vi "picturebox.vi"(8 "s":string, 11 "PictureBox":refnum<k24>(container)) -> ()   [LabVIEW 2024]
uses:
  System.Drawing
  System.Windows.Forms
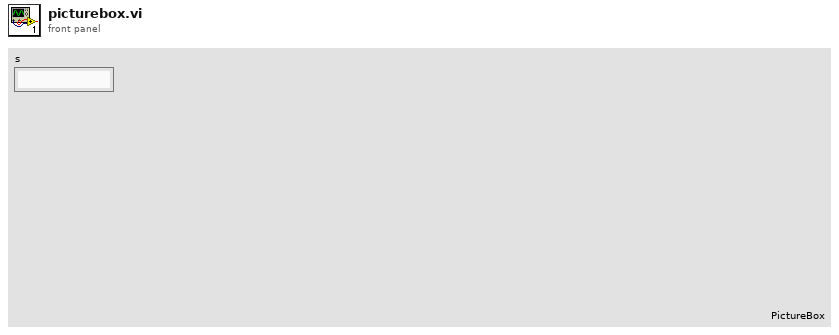
[diagram p1: front panel]
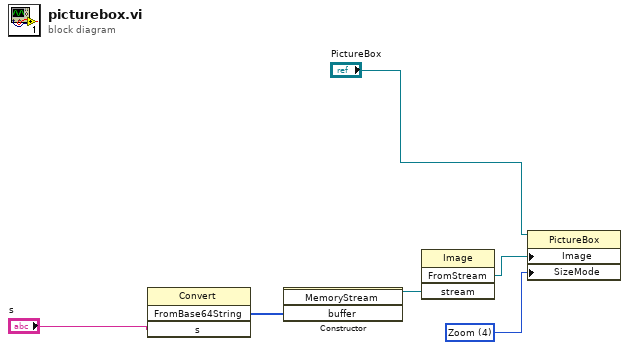
[diagram p0: block diagram]
diagram:
  w3 = 4 items=["Normal", "StretchImage", "AutoSize", "CenterImage", "Zoom"] ("SizeMode")
  n1 = invoke class="Convert" method="FromBase64String"("s"="s") -> ("FromBase64String"=w6:u8[])  [unwired: 3 in, 3 out]
  n2 = constructor class="MemoryStream"("buffer"=w6) -> (reference out=w5:refnum<k24>)  [unwired: 3 in, 3 out]
  n3 = invoke class="Image" method="FromStream"("stream"=w5) -> ("FromStream"=w4:refnum<k24>)  [unwired: 3 in, 3 out]
  n4 = property class="PictureBox"(reference="PictureBox", "Image"=w4, "SizeMode"=w3) -> ()  [unwired: 1 in, 2 out]
